vi "set_img_info.vi"(8 "Error in":errorcluster caption="Error in (no error)", 10 "Height (in)":i32, 11 "Width (in)":i32) -> (0 "Error out":errorcluster, 2 "Height (out)":i32, 3 "Width (out)":i32, 4 "Set IMG Parameters Time (ms)":dbl)   [LabVIEW 2018]
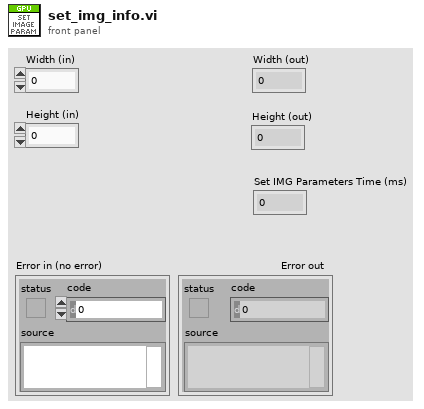
[diagram p1: front panel]
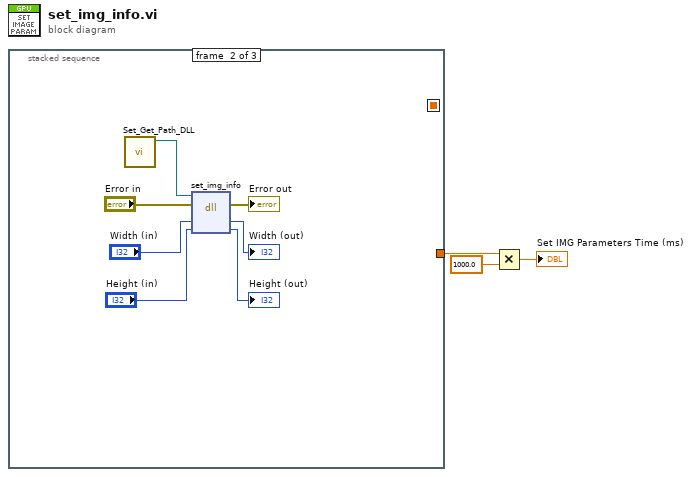
[diagram p0: block diagram]
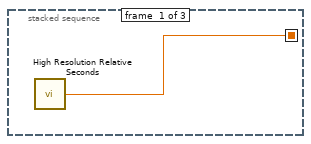
[diagram p2: hidden frame]
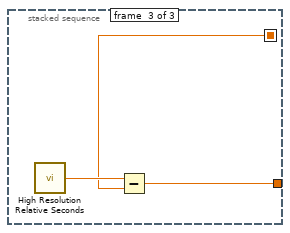
[diagram p3: hidden frame]
diagram:
  n1 = stacked-sequence {
    seq-local: [w4 _ _] -> [_ _ w12]
    tunnel: [_ _ w13] -> w3
    frame #0 {
      n2 = call <vilib>:"High Resolution Relative Seconds.vi"() -> ("relative seconds"=w4:dbl)
    }
    frame #1 {
      n3 = call "Set_Get_Path_DLL.vi"() -> ("path DLL Out"=w5:path)  [unwired: 11 in]
      n4 = dll-call lib="C:/Users/AUTIS/Documents/TFG/Proyecto/Visual Studio/SR_GPU_TOOLKIT_INIT/x64/Release/SR_GPU_TOOLKIT.dll" fn="set_img_info"(path in=w5, error in="Error in", "width"="Width (in)", "height"="Height (in)") -> (error out=→"Error out":errorcluster, "width"=→"Width (out)":i32, "height"=→"Height (out)":i32)  [unwired: 2 in, 1 out]
    }
    frame #2 {
      n5 = call <vilib>:"High Resolution Relative Seconds.vi"() -> ("relative seconds"=w14:dbl)
      n6 = Subtract(x=w14, y=w12) -> (x-y=w13:dbl)
    }
  }
  n7 = Multiply(x=w3, y=1000.0) -> (x*y=→"Set IMG Parameters Time (ms)":dbl)
